vi "Get Base Command.vi"(8 "error in (no error)":errorcluster, 11 "User Defined Write in":refnum<class "User Defined Write.lvclass">) -> (0 "error out":errorcluster, 2 "Base Command":string, 3 "User Defined Write out":refnum<class "User Defined Write.lvclass">)   [LabVIEW 2023, in "HAF.lvlib" / "User Defined Write.lvclass"]
doc: "Returns the base command whch is used to build up the overall command string – parameters will be added to this as necessary.  The framework will add the line terminator \\n.\n\nSubclasses MUST override this member and must not add a line terminator on the end of the command; on this class an error is returned."
uses:
  User Defined Write.lvclass
  User Defined Write.lvclass/User Defined Write.ctl
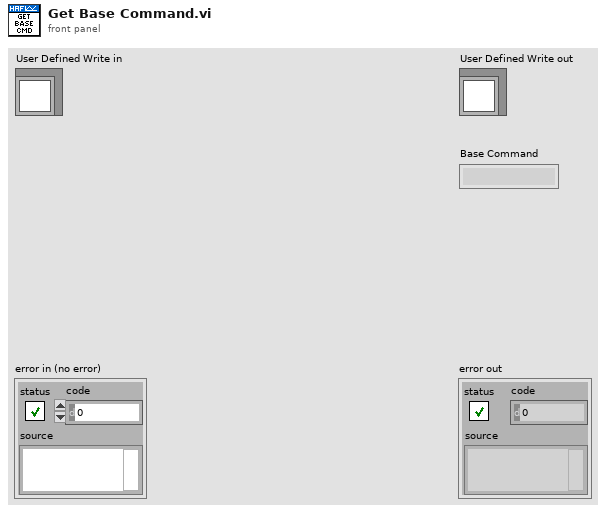
[diagram p1: front panel]
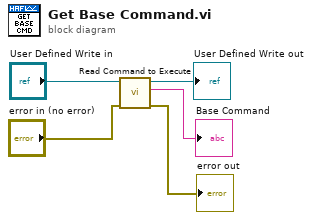
[diagram p0: block diagram]
diagram:
  n1 = call-dynamic "Read Command to Execute.vi"("error in (no error)"="error in (no error)", "User Defined Write in"="User Defined Write in") -> ("error out"=→"error out":errorcluster, "Command to Execute"=→"Base Command":string, "User Defined Write out"=→"User Defined Write out":refnum<class "User Defined Write.lvclass">)  [unwired: 7 in]
